vi "sensorcheckcolour.vi"   [LabVIEW 2013, in "mit2.lvrbt"]
uses:
  mit2.lvrbt
  <vilib>/NXT/Hardware/Plugins/Tetrix DC Motor/TetrixDCMotorAddress.ctl
  <vilib>/NXT/Block Support/NXT_InputPort.ctl
  <vilib>/NXT/Dual Mode Library/Sensors/Color_Detector.vi
  <vilib>/NXT/NXTIO Xnodes/NXTIONodeSubVIs/TETRIX IO Move DC Motors.vi
  <vilib>/NXT/NXTIO Xnodes/NXTIONodeSubVIs/TETRIX IO Stop DC Motors.vi
  <vilib>/NXT/NXTIO Xnodes/AddressXNode/NXTIOAddress.xnode
  <vilib>/NXT/Subs/LVHSConnector.ctl
  <vilib>/NXT/NXTIO Xnodes/NXTIOXNode/NXTIO.xnode
  <vilib>/NXT/LegoClasses/BrickReference/BrickReference.lvclass
types:
  T1 = typedef "TetrixDCMotorAddress.ctl" = i32
  T2 = cluster{"TetrixDCMotor":T1, "TetrixDCMotor 2":T1}
  T3 = typedef "NXT_InputPort.ctl" = u32
  T4 = typedef "LVHSConnector.ctl" = refnum<class "BrickReference.lvclass">
  T5 = typedef "ColorSensorColors.ctl" = enum16{"No Color", "Black", "Blue", "Green", "Yellow", "Red", "White", "Brown"}
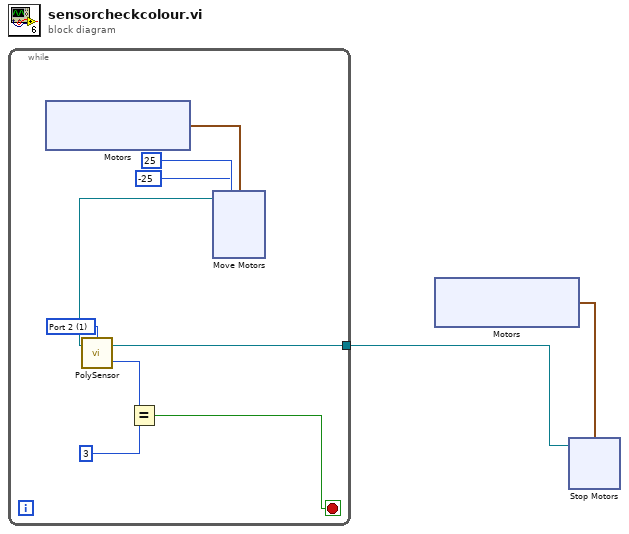
[diagram p0: block diagram]
diagram:
  n1 = while {
    tunnel: [w9] -> w2
    stop <- w3 stop-if-true
    w4 = T3 1 items=["Port 1", "Port 2", "Port 3", "Port 4"] ("Port (Port 3)")
    n2 = xnode "Motors"() -> ("Motor"=w11:cluster{"TetrixDCMotor":T1, "TetrixDCMotor":T1})
    n3 = xnode "Move Motors"("Power/Speed 2"=i8 -25, "Power/Speed 1"=i8 25, "Motors"=w11) -> ("NXT/EV3"=w10:T4)  [unwired: 1 in]
    n4 = call-poly <vilib>:"PolySensor.vi"("NXT/EV3"=w10, "Port (Port 3)"=w4) -> ("Detected Color"=w6:T5, "NXT/EV3"=w9:T4)  [unwired: 1 in]
    n5 = Equal?(x=w6, y=3) -> (x = y?=w3:bool)
  }
  n6 = xnode "Motors"() -> ("Motor"=w1:cluster{"TetrixDCMotor":T1, "TetrixDCMotor":T1})
  n7 = xnode "Stop Motors"("Motors"=w1, "NXT/EV3"=w2) -> ()  [unwired: 1 out]
